vi "omicron-pressure-logger-v2017-03-14-problems.vi"() -> ()   [LabVIEW 2016]
uses:
  <vilib>/addons/h5labview2/file/H5Fmode.ctl
  <vilib>/NI/Modbus Library/API/Wrapper/Create Serial Master.vi
  <vilib>/NI/Modbus Library/API/Master/Modbus Master.lvclass
  <vilib>/NI/Modbus Library/API/Wrapper/API Main.lvlib
  <vilib>/addons/h5labview2/file/H5F.lvlib
  <vilib>/addons/h5labview2/dataset/H5D.lvlib
panel:
  out "lt":sgl format="%_3e"
  in  "quit":bool
  out "Waveform Chart":dynamicdata(graph)
  out "oil pump":sgl
  out "prep":sgl caption="PREP" format="%_3e"
  # "(mbar)"
  # "(mbar)"
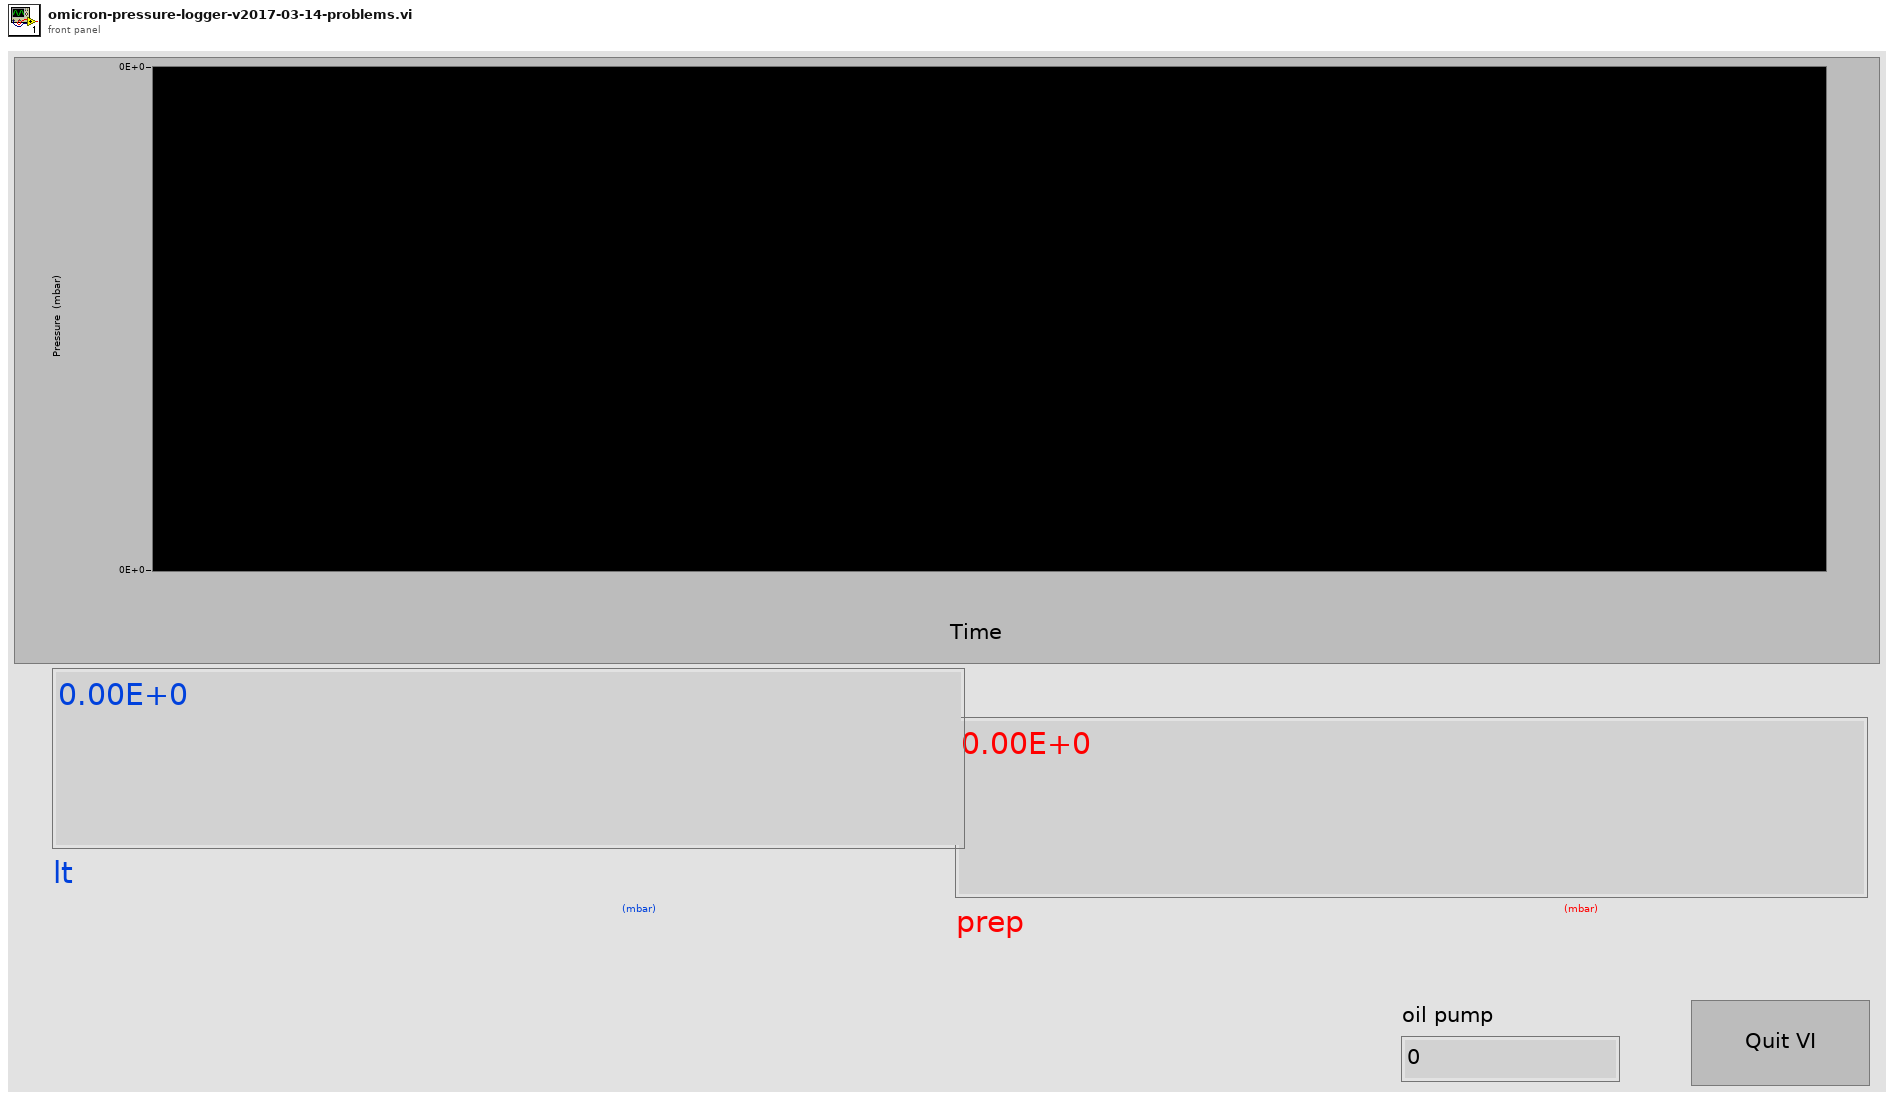
[diagram p1: front panel]
types:
  T1 = enum16{"open", "replace", "create", "open or create", "replace or create", "replace or create with confirmation"}
  T2 = typedef "H5F.lvlib/H5Fmode.ctl" = enum16{"read-only", "read-write", "overwrite", "create new", "open or create"}
  T3 = cluster{"timestamp":timestamp, "prep":sgl, "lt":sgl, "oil pump":sgl}
  T4 = typedef "hid_t.ctl" = i32
  T5 = cluster{"timestamp":timestamp, "prep":sgl, "lt":sgl, "oil pump":sgl}[]
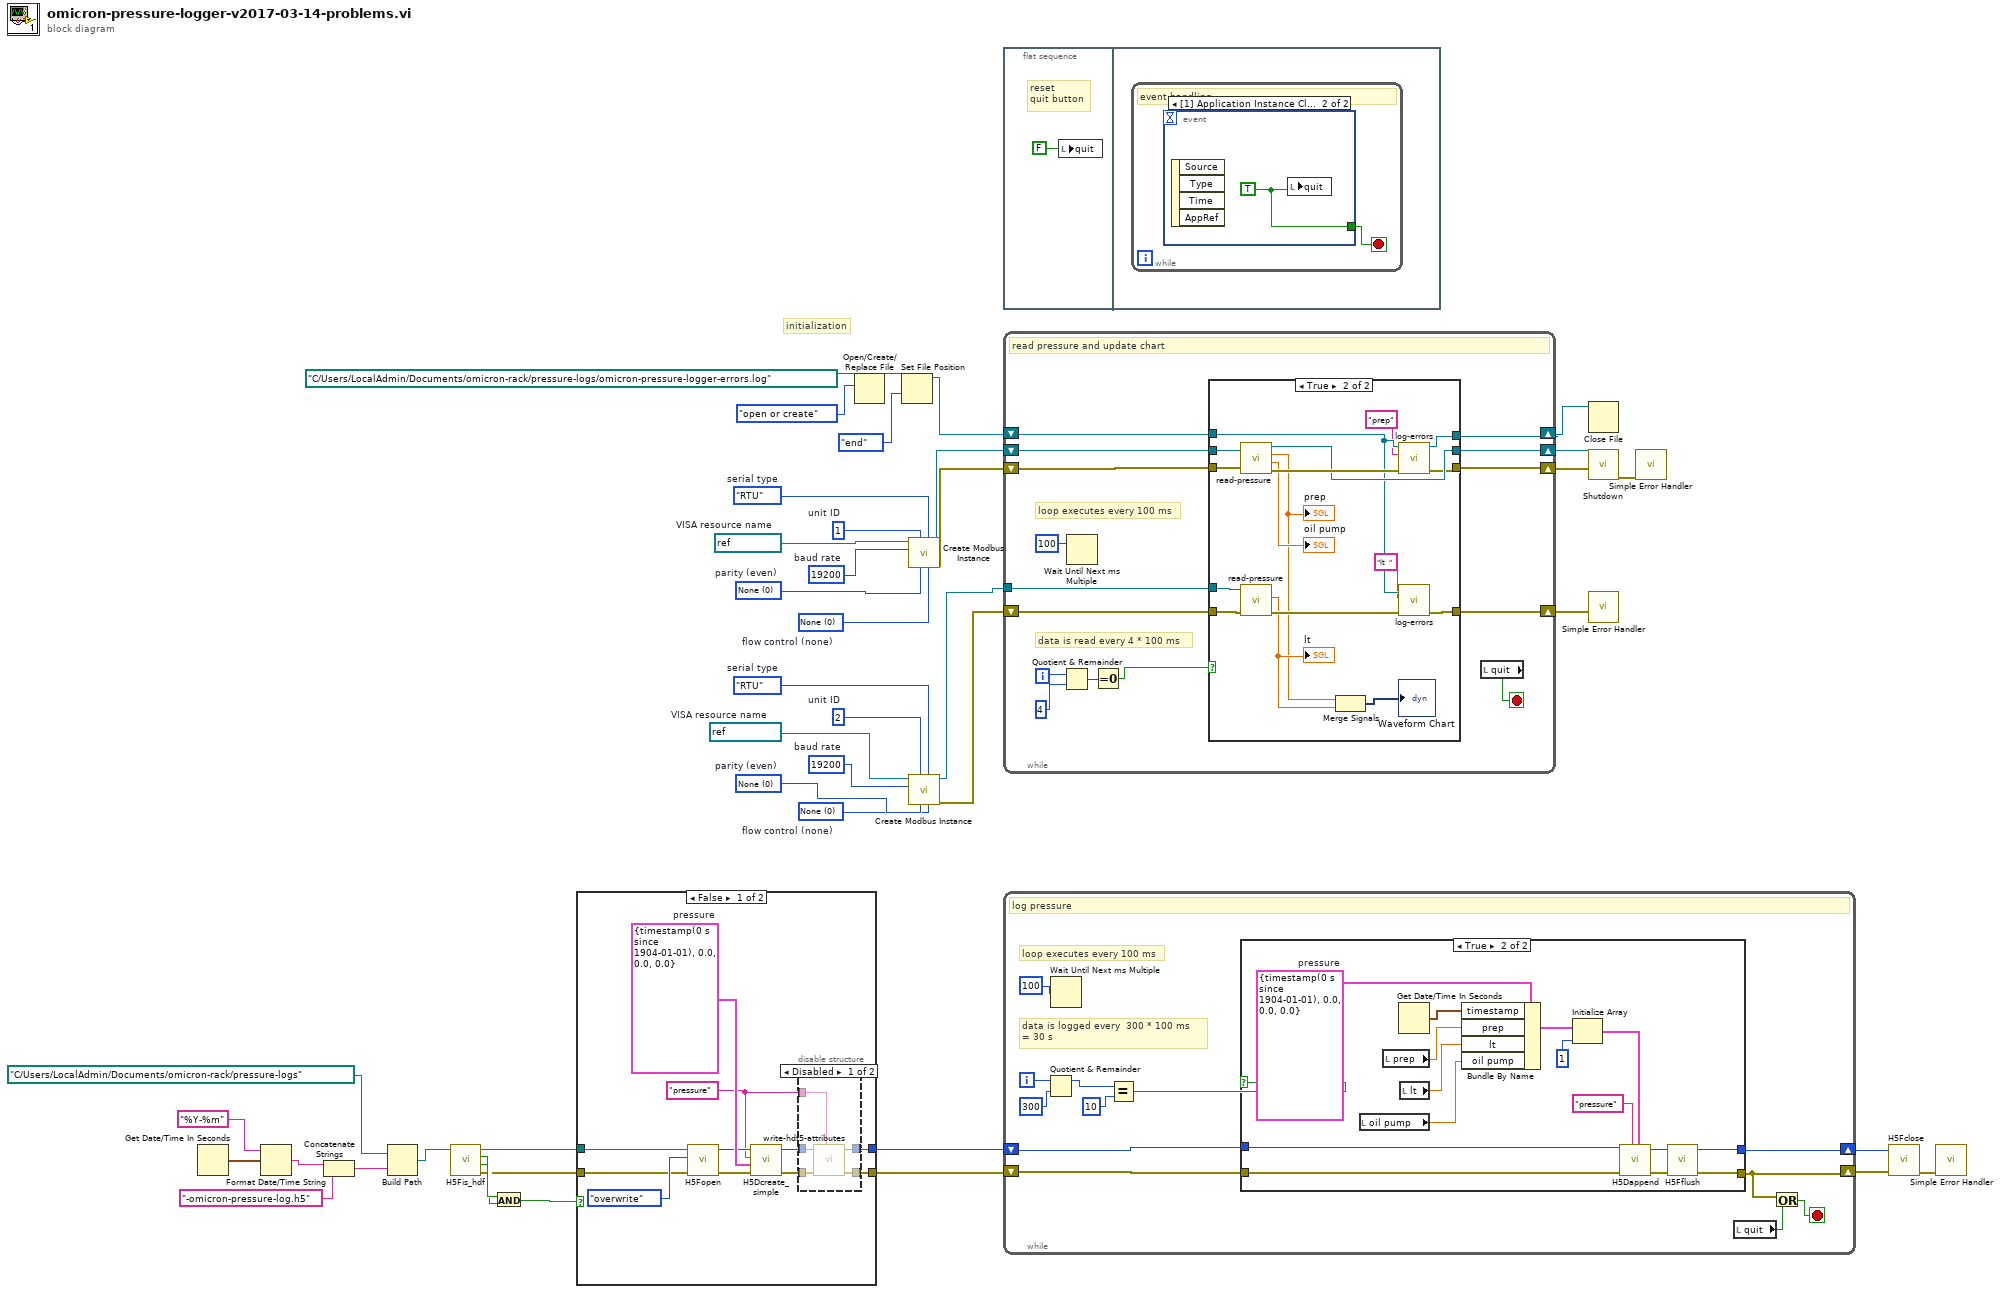
[diagram p0: block diagram]
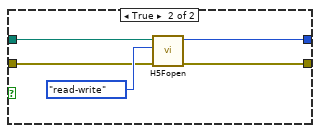
[diagram p3: hidden frame]
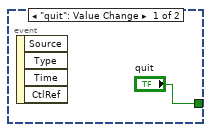
[diagram p4: hidden frame]
diagram:
  w18 = u16 0 items=["None", "XON/XOFF", "RTS/CTS", "XON/XOFF & RTS/CTS", "DTR/DSR", "XON/XOFF & DTR/DSR"]  # flow control (none)
  w19 = u16 0 items=["None", "Odd", "Even", "Mark", "Space"]  # parity (even)
  w22 = u32 19200  # baud rate
  w23 = refnum<visa-resource-name> "COM12"  # VISA resource name
  w21 = u8 2  # unit ID
  w20 = enum16{"RTU", "ASCII"}."RTU"  # serial type
  w33 = u16 0 items=["None", "XON/XOFF", "RTS/CTS", "XON/XOFF & RTS/CTS", "DTR/DSR", "XON/XOFF & DTR/DSR"]  # flow control (none)
  w34 = u16 0 items=["None", "Odd", "Even", "Mark", "Space"]  # parity (even)
  w37 = u32 19200  # baud rate
  w38 = refnum<visa-resource-name> "COM11"  # VISA resource name
  w36 = u8 1  # unit ID
  w35 = enum16{"RTU", "ASCII"}."RTU"  # serial type
  # "initialization"
  n1 = Get Date/Time In Seconds() -> (seconds since 1Jan1904=w14:timestamp)
  n2 = Format Date/Time String(time format string (%c)="%Y-%m", seconds (now)=w14) -> (date/time string=w12:string)  [unwired: 1 in]
  n3 = Concatenate Strings(w12, "-omicron-pressure-log.h5" ("string")) -> (w9:string)
  n4 = Build Path(base path=path "C:/Users/LocalAdmin/Documents/omicron-rack/pressure-logs" ("path"), name or relative path=w9) -> (appended path=w8:path)
  n5 = call <vilib>:"H5Fis_hdf.vi"("path in"=w8) -> ("error out"=w1:errorcluster, "valid?"=w6:bool, "exists?"=w7:bool, "path out"=w4:path)  [unwired: 7 in]
  n6 = And(x=w7, y=w6) -> (x .and. y?=w5:bool)
  n7 = case shown="False" w5 {
    tunnel: w4 -> [w53 w63]
    tunnel: [w46 w60] -> w3
    tunnel: [w45 w61] -> w2
    tunnel: w1 -> [w52 w62]
    frame False {
      w44 = "pressure" ("name")
      w51 = T3 {"timestamp"=timestamp(0 s since 1904-01-01), "prep"=0.0, "lt"=0.0, "oil pump"=0.0}  # pressure
      n8 = call <vilib>:"H5Fopen.vi"("error in (no error)"=w52, "mode (read-only)"=H5Fmode."overwrite", "path"=w53) -> ("error out"=w49:errorcluster, "ref out"=w50:T4)  [unwired: 7 in]
      n9 = call <vilib>:"H5Dcreate_simple.vi"("error in (no error)"=w49, "type in"=w51, "name"=w44, "ref in"=w50) -> ("error out"=w47:errorcluster, "dset out"=w48:T4)  [unwired: 6 in]
      n10 = disable-structure shown="Disabled" {
        disable-tunnel: w48 -> [w59 _]
        disable-tunnel: w47 -> [w58 _]
        disable-tunnel: [w57 _] -> w46
        disable-tunnel: [w56 _] -> w45
        disable-tunnel: w44 -> [w55 _]
        frame Disabled {
          n11 = call "write-hdf5-attributes.vi"("name"=w55, "error in (no error)"=w58, "ref in"=w59) -> ("error out"=w56:errorcluster, "ref out"=w57:i32)  [unwired: 7 in]
        }
        frame Enabled {
        }
      }
    }
    frame True {
      n12 = call <vilib>:"H5Fopen.vi"("error in (no error)"=w62, "mode (read-only)"=H5Fmode."read-write", "path"=w63) -> ("error out"=w61:errorcluster, "ref out"=w60:T4)  [unwired: 7 in]
    }
  }
  n13 = Open/Create/Replace File(file path (use dialog)=path "C:/Users/LocalAdmin/Documents/omicron-rack/pressure-logs/omicron-pressure-logger-errors.log" ("Path"), operation (0:open)=T1."open or create") -> (refnum out=w30:refnum<file>)  [unwired: 4 in, 2 out]
  n14 = Set File Position(refnum=w30, from (0:start)=enum16{"start", "end", "current"}."end") -> (refnum out=w39:refnum<file>)  [unwired: 2 in, 1 out]
  n15 = call-poly <vilib>:"Create Modbus Instance.vi"("flow control (none)"=w33, "serial type"=w35, "parity (even)"=w34, "unit ID"=w36, "baud rate"=w37, "VISA resource name"=w38) -> ("error out"=w42:errorcluster, "serial master instance"=w43:refnum<class "Modbus Master.lvclass">)  [unwired: 4 in]
  n16 = call-poly <vilib>:"Create Modbus Instance.vi"("flow control (none)"=w18, "serial type"=w20, "parity (even)"=w19, "unit ID"=w21, "baud rate"=w22, "VISA resource name"=w23) -> ("error out"=w16:errorcluster, "serial master instance"=w17:refnum<class "Modbus Master.lvclass">)  [unwired: 4 in]
  n17 = flat-sequence {
    frame #0 {
      # "reset\nquit button"
      n18 = local write "quit"(FALSE) -> ()
    }
    frame #1 {
      n19 = while {
        stop <- w66 stop-if-true
        # "event handling"
        n20 = event shown="[1] Application Instance Close" {
          selector: _ -> [_ _]
          dyn-events: _ -> [_ _]
          timeout: _ -> [_ _]
          tunnel: ["quit" w68] -> w66
          event "quit": Value Change {
            n21 = event-data() -> ()  [unwired: 1 in, 4 out]
          }
          event Application Instance Close {
            w68 = TRUE
            n22 = event-data() -> ()  [unwired: 1 in, 4 out]
            n23 = local write "quit"(w68) -> ()
          }
        }
      }
    }
  }
  n24 = while {
    shift-right: [w73] -> w41
    shift-left: w43 -> [w76]
    shift-right: [w72] -> w40
    shift-left: w42 -> [w75]
    shift-right: [w74] -> w28
    shift-left: w39 -> [w77]
    tunnel: w17 -> [w71]
    shift-right: [w69] -> w15
    shift-left: w16 -> [w70]
    i -> [w78]
    stop <- w83 stop-if-true
    # "data is read every 4 * 100 ms"
    # "loop executes every 100 ms"
    # "read pressure and update chart"
    n25 = Quotient & Remainder(x=w78, y=4) -> (x-y*floor(x/y)=w80:i32)  [unwired: 1 out]
    n26 = Wait Until Next ms Multiple(millisecond multiple=u32 100 ("milliseconds to wait")) -> ()  [unwired: 1 out]
    n27 = Equal To 0?(x=w80) -> (x = 0?=w79:bool)
    n28 = case shown="True" w79 {
      tunnel: w77 -> [w87 w93]
      tunnel: w76 -> [w85 w102]
      tunnel: w75 -> [w86 w101]
      tunnel: [w87 w97] -> w74
      tunnel: [w86 w98] -> w72
      tunnel: [w85 w99] -> w73
      tunnel: w71 -> [_ w96]
      tunnel: w70 -> [w84 w95]
      tunnel: [w84 w94] -> w69
      frame False {
      }
      frame True {
        n29 = call "read-pressure.vi"("error in"=w101, "Modbus instance in"=w102) -> ("error out"=w104:errorcluster, "Pirani"=→"oil pump":sgl, "Ion Gauge Pressure"=w88:sgl, "Modbus instance out"=w99:refnum<class "Modbus Master.lvclass">)  [unwired: 6 in]
        "prep" <- w88
        n30 = call "read-pressure.vi"("error in"=w95, "Modbus instance in"=w96) -> ("error out"=w100:errorcluster, "Ion Gauge Pressure"=w89:sgl)  [unwired: 6 in, 2 out]
        "lt" <- w89
        n31 = Merge Signals(w88, w89) -> (→"Waveform Chart":dynamicdata)
        n32 = call "log-errors.vi"("error in (no error)"=w104, "device"="prep", "refnum in"=w93) -> ("error out"=w98:errorcluster, "refnum out"=w97:refnum<file>)  [unwired: 7 in]
        n33 = call "log-errors.vi"("error in (no error)"=w100, "device"="lt  ", "refnum in"=w93) -> ("error out"=w94:errorcluster)  [unwired: 7 in, 1 out]
      }
    }
    n34 = local read "quit"() -> (w83:bool)
  }
  n35 = while {
    shift-right: [w109] -> w26
    shift-left: w3 -> [w111]
    shift-right: [w107] -> w25
    shift-left: w2 -> [w110]
    i -> [w113]
    stop <- w108 stop-if-true
    # "data is logged every  300 * 100 ms\n= 30 s"
    # "loop executes every 100 ms"
    # "log pressure"
    n36 = Quotient & Remainder(x=w113, y=300) -> (x-y*floor(x/y)=w106:i32)  [unwired: 1 out]
    n37 = Wait Until Next ms Multiple(millisecond multiple=u32 100 ("milliseconds to wait")) -> ()  [unwired: 1 out]
    n38 = Equal?(x=w106, y=10) -> (x = y?=w112:bool)
    n39 = case shown="True" w112 {
      tunnel: w111 -> [w118 w125]
      tunnel: w110 -> [w117 w124]
      tunnel: [w118 w119] -> w109
      tunnel: [w117 w121] -> w107
      frame False {
      }
      frame True {
        w132 = T3 {"timestamp"=timestamp(0 s since 1904-01-01), "prep"=0.0, "lt"=0.0, "oil pump"=0.0}  # pressure
        n40 = local read "oil pump"() -> (w130:sgl)
        n41 = local read "prep"() -> (w131:sgl)
        n42 = Get Date/Time In Seconds() -> (seconds since 1Jan1904=w133:timestamp)
        n43 = local read "lt"() -> (w122:sgl)
        n44 = Bundle By Name(cluster=w132, "timestamp"=w133, "prep"=w131, "lt"=w122, "oil pump"=w130) -> (w128:T3)
        n45 = Initialize Array(w128, 1 ("dimension size")) -> (w126:T5)
        n46 = call <vilib>:"H5Dappend.vi"("dataset name"="pressure" ("name"), "error in (no error)"=w124, "data"=w126, "ref in"=w125) -> ("error out"=w123:errorcluster, "ref out"=w120:T4)  [unwired: 4 in, 2 out]
        n47 = call <vilib>:"H5Fflush.vi"("error in (no error)"=w123, "ref in"=w120) -> ("error out"=w121:errorcluster, "ref out"=w119:T4)  [unwired: 8 in]
      }
    }
    n48 = local read "quit"() -> (w116:bool)
    n49 = Or(x=w107, y=w116) -> (x .or. y?=w108:bool)
  }
  n50 = Close File(refnum=w28) -> ()  [unwired: 1 in, 2 out]
  n51 = call-dynamic "Shutdown.vi"("error in"=w40, "Modbus master in"=w41) -> ("error out"=w24:errorcluster)  [unwired: 9 in]
  n52 = call <vilib>:"Simple Error Handler.vi"("error in (no error)"=w15) -> ()  [unwired: 4 in, 5 out]
  n53 = call <vilib>:"Simple Error Handler.vi"("error in (no error)"=w24) -> ()  [unwired: 4 in, 5 out]
  n54 = call <vilib>:"H5Fclose.vi"("error in (no error)"=w25, "ref"=w26) -> ("error out"=w27:errorcluster)  [unwired: 9 in]
  n55 = call <vilib>:"Simple Error Handler.vi"("error in (no error)"=w27) -> ()  [unwired: 4 in, 5 out]
